vi "lab3.vi"() -> ()   [LabVIEW 2020]
panel:
  out "XY Graph":cluster{"X":dbl[], "Y":dbl[]}[](graph)
  out "Path":path
  out "VCt":dbl[](array[numeric])
  out "It":dbl[](array[numeric])
  in  "VISA resource name 2":refnum<visa-resource-name>
  in  "Manual Range (0)":dbl
  in  "Function (0: Voltage DC)":i32(ring) items=[" Voltage DC", "Voltage AC", "Current DC", "Current AC", "Resistance", "4-wire Resistance", "Diode", "Capacitance", "Temperature", "Continuity", "Frequency", "Period", "Voltage Ratio", "Digitize Voltage", "Digitize Current"]
  in  "Auto Range (T: Enable)":bool=TRUE
  in  "Auto Zero (0: Enable)":u32(ring) items=["Enable", "Disable", "Once"]
  out "Measurements":dbl
  in  "VISA resource name":refnum<visa-resource-name>
  in  "Reset? (T: Yes)":bool=TRUE
  out "VISA resource name out":refnum<visa-resource-name>
  in  "Output State":u16(ring) items=["OFF", "ON"]
  in  "Output Current":dbl=1.0
  out "Measured Voltage":sgl
  out "Measured Current":sgl
  in  "step(VC)":dbl
  in  "max(VC)":dbl
  in  "min(VC)":dbl
  in  "step(VB)":dbl
  in  "max(VB)":dbl
  in  "min(VB)":dbl
  out "VC":dbl[][](array[numeric])
  out "VB":dbl[](array[numeric])
  out "I":dbl[][](array[numeric])
  # "电压源 2231A-30-A"
  # "万用表 DMM6500"
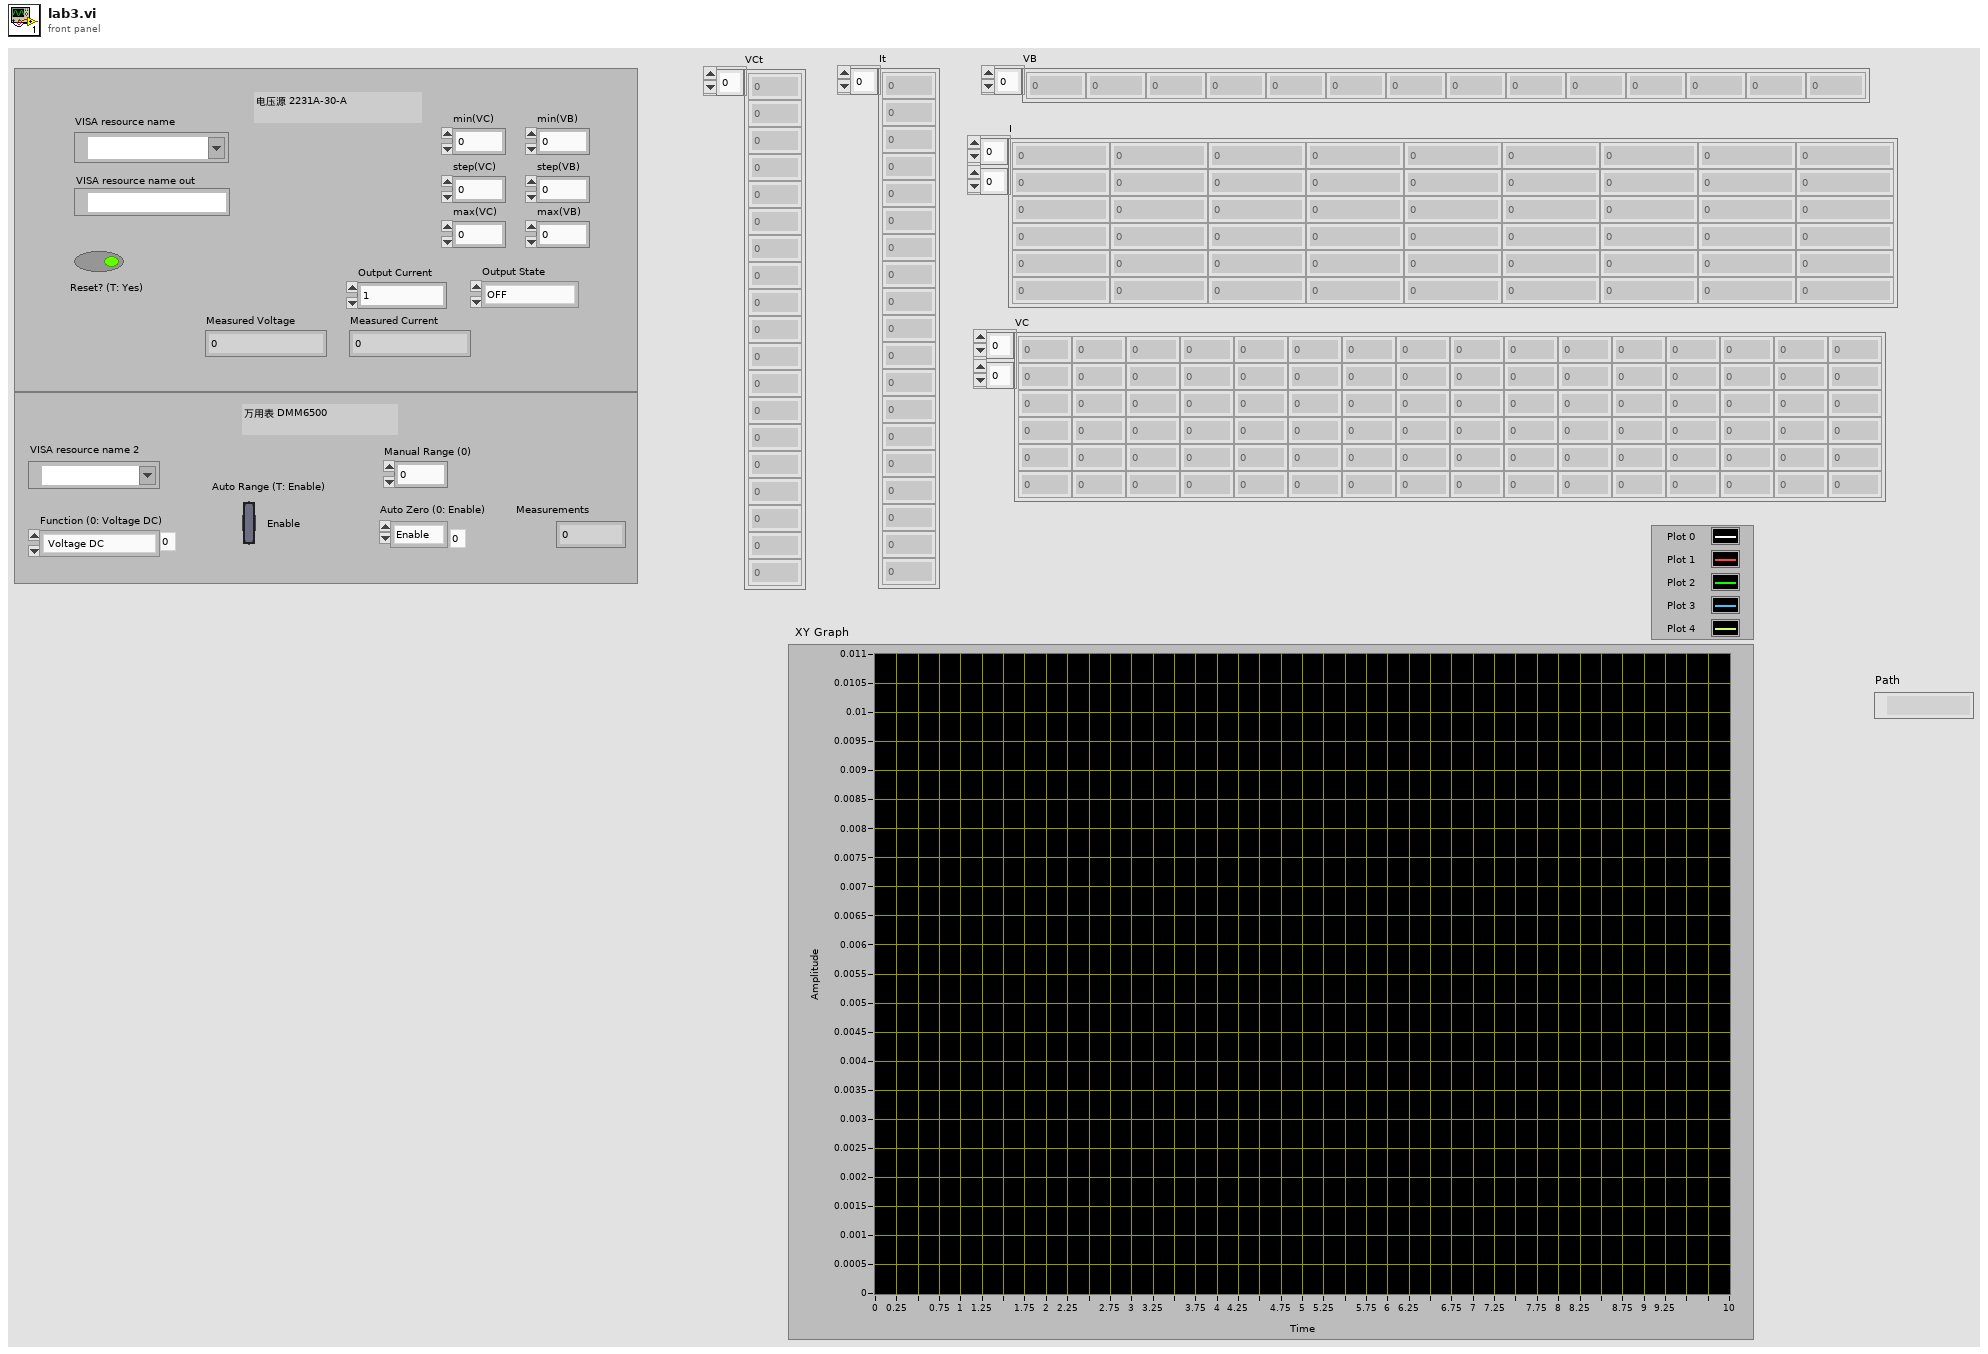
[diagram p1: front panel]
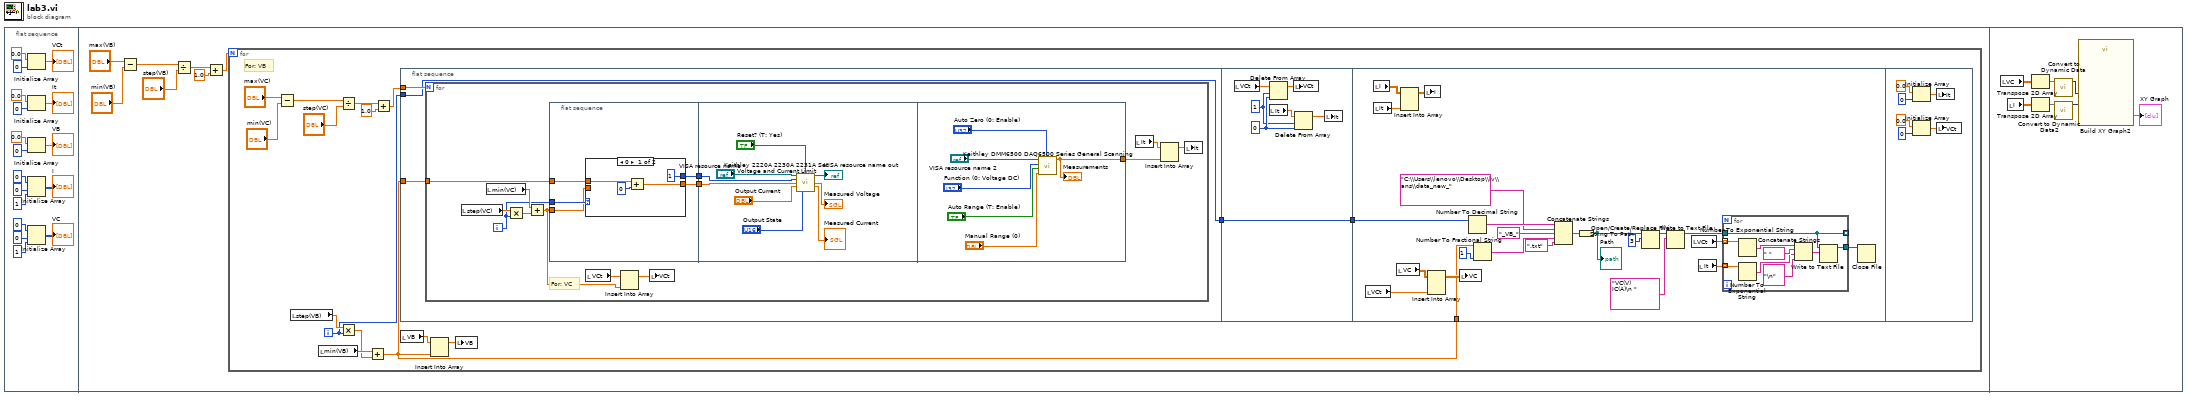
[diagram p0: block diagram]
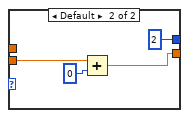
[diagram p2: hidden frame]
diagram:
  n1 = flat-sequence {
    frame #0 {
      n2 = Initialize Array(0.0 ("element"), 0 ("dimension size")) -> (→"VCt":dbl[])
      n3 = Initialize Array(0.0 ("element"), 0 ("dimension size")) -> (→"It":dbl[])
      n4 = Initialize Array(0.0 ("element"), 0 ("dimension size")) -> (→"VB":dbl[])
      n5 = Initialize Array(0, 0, 1) -> (→"I":i32[][])
      n6 = Initialize Array(0, 0, 1) -> (→"VC":i32[][])
    }
    frame #1 {
      n7 = Subtract(x="max(VB)", y="min(VB)") -> (x-y=w22:dbl)
      n8 = Divide(x=w22, y="step(VB)") -> (x/y=w20:dbl)
      n9 = Add(x=w20, y=1.0) -> (x+y=w18:dbl)
      n10 = for {
        N: w18 -> [_]
        i -> [w27]
        # "For: VB"
        n11 = Subtract(x="max(VC)", y="min(VC)") -> (x-y=w38:dbl)
        n12 = local read "step(VB)"() -> (w33:dbl)
        n13 = local read "min(VB)"() -> (w34:dbl)
        n14 = Divide(x=w38, y="step(VC)") -> (x/y=w36:dbl)
        n15 = Multiply(x=w33, y=w27) -> (x*y=w32:dbl)
        n16 = Add(x=w34, y=w32) -> (x+y=w28:dbl)
        n17 = Add(x=w36, y=1.0) -> (x+y=w31:dbl)
        n18 = flat-sequence {
          tunnel: w31 -> [w43]
          tunnel: w28 -> [w42]
          tunnel: w27 -> [w41]
          tunnel: [w41] -> w26
          tunnel: w26 -> [w85]
          tunnel: [w85] -> w25
          tunnel: w28 -> [w98]
          tunnel: w25 -> [w108]
          frame #0 {
            n19 = for {
              N: w43 -> [_]
              tunnel: w42 -> [w49]
              i -> [w50]
              # "For: VC"
              n20 = local read "step(VC)"() -> (w55:dbl)
              n21 = local read "min(VC)"() -> (w56:dbl)
              n22 = Multiply(x=w55, y=w50) -> (x*y=w54:dbl)
              n23 = Add(x=w56, y=w54) -> (x+y=w44:dbl)
              n24 = flat-sequence {
                tunnel: w50 -> [w61]
                tunnel: w49 -> [w60]
                tunnel: w44 -> [w59]
                tunnel: [w58] -> w48
                tunnel: [w57] -> w47
                tunnel: w48 -> [w71]
                tunnel: w47 -> [w70]
                tunnel: [w79] -> w51
                frame #0 {
                  n25 = case shown="0" w61 {
                    tunnel: w60 -> [w65 _]
                    tunnel: [w63 w68] -> w58
                    tunnel: w59 -> [_ w67]
                    tunnel: [1 2] -> w57
                    frame 0 {
                      n26 = Add(x=w65, y=0) -> (x+y=w63:dbl)
                    }
                    frame Default {
                      n27 = Add(x=w67, y=0) -> (x+y=w68:dbl)
                    }
                  }
                }
                frame #1 {
                  n28 = call "Keithley 2220A 2230A 2231A Set Voltage and Current Limit.vi"("VISA resource name"="VISA resource name", "Reset? (T: Yes)"="Reset? (T: Yes)", "Channel Control"=w70, "Supply Voltage"=w71, "Output Current"="Output Current", "Output State"="Output State") -> ("VISA resource name out"=→"VISA resource name out":refnum<visa-resource-name>, "Measured Voltage"=→"Measured Voltage":sgl, "Measured Current"=→"Measured Current":sgl)  [unwired: 6 in, 1 out]
                }
                frame #2 {
                  n29 = call "Keithley DMM6500 DAQ6500 Series General Scanning.vi"("Auto Zero (0: Enable)"="Auto Zero (0: Enable)", "Manual Range (0)"="Manual Range (0)", "Auto Range (T: Enable)"="Auto Range (T: Enable)", "Function (0: Voltage DC)"="Function (0: Voltage DC)", "VISA resource name"="VISA resource name 2") -> ("Measurements"=w79:dbl)  [unwired: 6 in]
                  "Measurements" <- w79
                }
              }
              n30 = local read "VCt"() -> (w45:dbl[])
              n31 = Insert Into Array(array=w45, new element=w44) -> (w46:dbl[])  [unwired: 1 in]
              n32 = local write "VCt"(w46) -> ()
              n33 = local read "It"() -> (w53:dbl[])
              n34 = Insert Into Array(array=w53, new element=w51) -> (w52:dbl[])  [unwired: 1 in]
              n35 = local write "It"(w52) -> ()
            }
          }
          frame #1 {
            w86 = 1
            w89 = 0
            n36 = local read "VCt"() -> (w90:dbl[])
            n37 = Delete From Array(array=w90, length=w86, index=w89) -> (array with subset deleted=w87:dbl[])  [unwired: 1 out]
            n38 = local read "It"() -> (w91:dbl[])
            n39 = local write "VCt"(w87) -> ()
            n40 = Delete From Array(array=w91, length=w86, index=w89) -> (array with subset deleted=w88:dbl[])  [unwired: 1 out]
            n41 = local write "It"(w88) -> ()
          }
          frame #2 {
            n42 = local read "VCt"() -> (w110:dbl[])
            n43 = local read "I"() -> (w111:dbl[][])
            n44 = local read "It"() -> (w109:dbl[])
            n45 = local read "VC"() -> (w114:dbl[][])
            n46 = Insert Into Array(array=w111, new element=w109) -> (w112:dbl[][])  [unwired: 2 in]
            n47 = local write "I"(w112) -> ()
            n48 = Insert Into Array(array=w114, new element=w110) -> (w113:dbl[][])  [unwired: 2 in]
            n49 = local write "VC"(w113) -> ()
            n50 = Number To Decimal String(number=w108) -> (decimal integer string=w106:string)  [unwired: 1 in]
            n51 = Number To Fractional String(number=w98, precision (6)=1) -> (F-format string=w99:string)  [unwired: 2 in]
            n52 = Concatenate Strings("C:\\Users\\lenovo\\Desktop\\lv\\ans\\data_new_", w106, "_VB_", w99, ".txt") -> (w104:string)
            n53 = String To Path(string=w104) -> (path=w102:path)
            "Path" <- w102
            n54 = Open/Create/Replace File(file path (use dialog)=w102, operation (0:open)=3) -> (refnum out=w94:refnum<file>)  [unwired: 4 in, 2 out]
            n55 = Write to Text File(file (use dialog)=w94, text="VC(V)             IC(A)\n ") -> (refnum out=w93:refnum<file>)  [unwired: 2 in, 2 out]
            n56 = local read "VCt"() -> (w95:dbl[])
            n57 = local read "It"() -> (w100:dbl[])
            n58 = for {
              tunnel: [w115] -> _ mode=indexing
              tunnel: [w123] -> w101
              tunnel: w100 -> [w122] mode=indexing
              tunnel: w95 -> [w121] mode=indexing
              tunnel: w93 -> [w115]
              n59 = Number To Exponential String(number=w121) -> (E-format string=w119:string)  [unwired: 3 in]
              n60 = Number To Exponential String(number=w122) -> (E-format string=w118:string)  [unwired: 3 in]
              n61 = Concatenate Strings(w119, " ", w118, "\n") -> (w117:string)
              n62 = Write to Text File(file (use dialog)=w115, text=w117) -> (refnum out=w123:refnum<file>)  [unwired: 2 in, 2 out]
            }
            n63 = Close File(refnum=w101) -> ()  [unwired: 1 in, 2 out]
          }
          frame #3 {
            n64 = Initialize Array(0.0 ("element"), 0 ("dimension size")) -> (w124:dbl[])
            n65 = Initialize Array(0.0 ("element"), 0 ("dimension size")) -> (w125:dbl[])
            n66 = local write "It"(w124) -> ()
            n67 = local write "VCt"(w125) -> ()
          }
        }
        n68 = local read "VB"() -> (w29:dbl[])
        n69 = Insert Into Array(array=w29, new element=w28) -> (w30:dbl[])  [unwired: 1 in]
        n70 = local write "VB"(w30) -> ()
      }
    }
    frame #2 {
      n71 = local read "VC"() -> (w134:dbl[][])
      n72 = local read "I"() -> (w136:dbl[][])
      n73 = Transpose 2D Array(2D array=w134) -> (transposed array=w133:dbl[][])
      n74 = Transpose 2D Array(2D array=w136) -> (transposed array=w135:dbl[][])
      n75 = call "Convert to Dynamic Data"("2D Array"=w133) -> ("Dynamic Data Type"=w131:dynamicdata)  [unwired: 3 in]
      n76 = call "Convert to Dynamic Data2"("2D Array"=w135) -> ("Dynamic Data Type"=w132:dynamicdata)  [unwired: 3 in]
      n77 = call "Build XY Graph2"("Y Input"=w132, "X Input"=w131) -> ("XY Graph"=→"XY Graph":cluster{"X":dbl[], "Y":dbl[]}[])  [unwired: 8 in, 1 out]
    }
  }
